vi "servo chB.vi"(0 "Servo Position (0 - 255)":u8(slide)=128 step=1 scale=0.0..255.0, 1 "Controller Daisy Chain Position (1 - 4)":u8=1, 4 "Enable Sync: Fast | Medium | Slow | None":string(combo)="None", 5 "Select Servo":string(combo)="Servo 1", 6 "Enum":enum16{"A", "B"}(ring), 7 "error in (no error)":errorcluster) -> (2 "error out":errorcluster)   [LabVIEW 2018]
uses:
  <vilib>/myRIO/Instrument Drivers/Onboard IO/I2C/typedefs/I2C User Configuration.ctl
  <vilib>/myRIO/Instrument Drivers/Onboard IO/I2C/typedefs/I2C Transfer Rate.ctl
  <vilib>/myRIO/Instrument Drivers/Onboard IO/I2C/typedefs/I2C Reference.ctl
  <vilib>/myRIO/Common/Instrument Driver Framework/Utilities/typedefs/myRIO Generic Hardware Reference.ctl
  <vilib>/myRIO/Common/Instrument Driver Framework/Utilities/typedefs/Hardware Version Enum.ctl
  <vilib>/myRIO/Common/Instrument Driver Framework/Utilities/typedefs/myRIO v1.0 Reference.ctl
  <vilib>/myRIO/Common/Instrument Driver Framework/Utilities/typedefs/Generic FPGA Reference.ctl
  <vilib>/myRIO/Common/Instrument Driver Framework/myRIO v1.0/I2C/typedefs/I2C Channels Enum.ctl
  <vilib>/myRIO/Instrument Drivers/Onboard IO/I2C/typedefs/I2C Configuration.ctl
  <vilib>/userdefined/High Color/nirio_resource_hc.ctl
  <vilib>/myRIO/Common/Instrument Driver Framework/Utilities/vis/Is FPGA Ref Available.vi
  <vilib>/myRIO/Common/Instrument Driver Framework/myRIO v1.0/I2C/vis/myRIO v1.1 Open I2C.vi
  <vilib>/myRIO/Instrument Drivers/Onboard IO/I2C/vis/Configure.vi
  <vilib>/myRIO/Instrument Drivers/Onboard IO/I2C/vis/Write.vi
  <vilib>/myRIO/Common/Instrument Driver Framework/Utilities/vis/Validate Channels.vi
  <vilib>/myRIO/Common/Instrument Driver Framework/myRIO v1.0/I2C/vis/myRIO v1.0 Reserve I2C.vi
  <vilib>/myRIO/Common/Instrument Driver Framework/myRIO v1.0/I2C/vis/myRIO v1.0 Build MUX Configuration I2C.vi
  <vilib>/myRIO/Common/Instrument Driver Framework/myRIO v1.0/Resource Manager/vis/myRIO v1.0 Reserve Channel List.vi
  <vilib>/myRIO/Common/Instrument Driver Framework/myRIO v1.0/Resource Manager/vis/myRIO v1.0 Create Configuration List.vi
  <vilib>/myRIO/Common/Instrument Driver Framework/myRIO v1.0/Resource Manager/vis/myRIO v1.0 Reserve Channel.vi
  <vilib>/myRIO/Common/Instrument Driver Framework/myRIO v1.0/Resource Manager/vis/myRIO v1.0 Unreserve Channel.vi
  <vilib>/myRIO/Common/Instrument Driver Framework/myRIO v1.0/Resource Manager/vis/myRIO v1.0 Build Mutex Name.vi
  <vilib>/Utility/VariantDataType/GetNumericInfo.vi
  <vilib>/Utility/error.llb/Error Cluster From Error Code.vi
  <vilib>/myRIO/Common/Instrument Driver Framework/myRIO v1.0/myRIO v1.1 Open.vi
  <vilib>/myRIO/Common/Instrument Driver Framework/Utilities/vis/IO Manager.vi
  <vilib>/myRIO/Common/Instrument Driver Framework/Utilities/vis/Configuration Manager.vi
  <vilib>/myRIO/Common/Instrument Driver Framework/myRIO v1.0/Resource Manager/vis/myRIO v1.0 Configure IO.vi
  <vilib>/myRIO/Common/Instrument Driver Framework/myRIO v1.0/myRIO v1.0 Close.vi
  <vilib>/myRIO/Common/Instrument Driver Framework/myRIO v1.0/I2C/vis/myRIO v1.0 Configure I2C.vi
  <vilib>/myRIO/Common/Instrument Driver Framework/myRIO v1.0/I2C/vis/myRIO v1.0 Write I2C.vi
  <vilib>/myRIO/Express VI/Onboard IO/I2C/I2C Express VI.xnode
  <vilib>/myRIO/Instrument Drivers/Onboard IO/I2C/vis/myRIO I2C Open.xnode
  <vilib>/myRIO/Instrument Drivers/Onboard IO/I2C/I2C.lvlib
panel:
  out "error out 2":errorcluster
  in  "error in (no error) 2":errorcluster
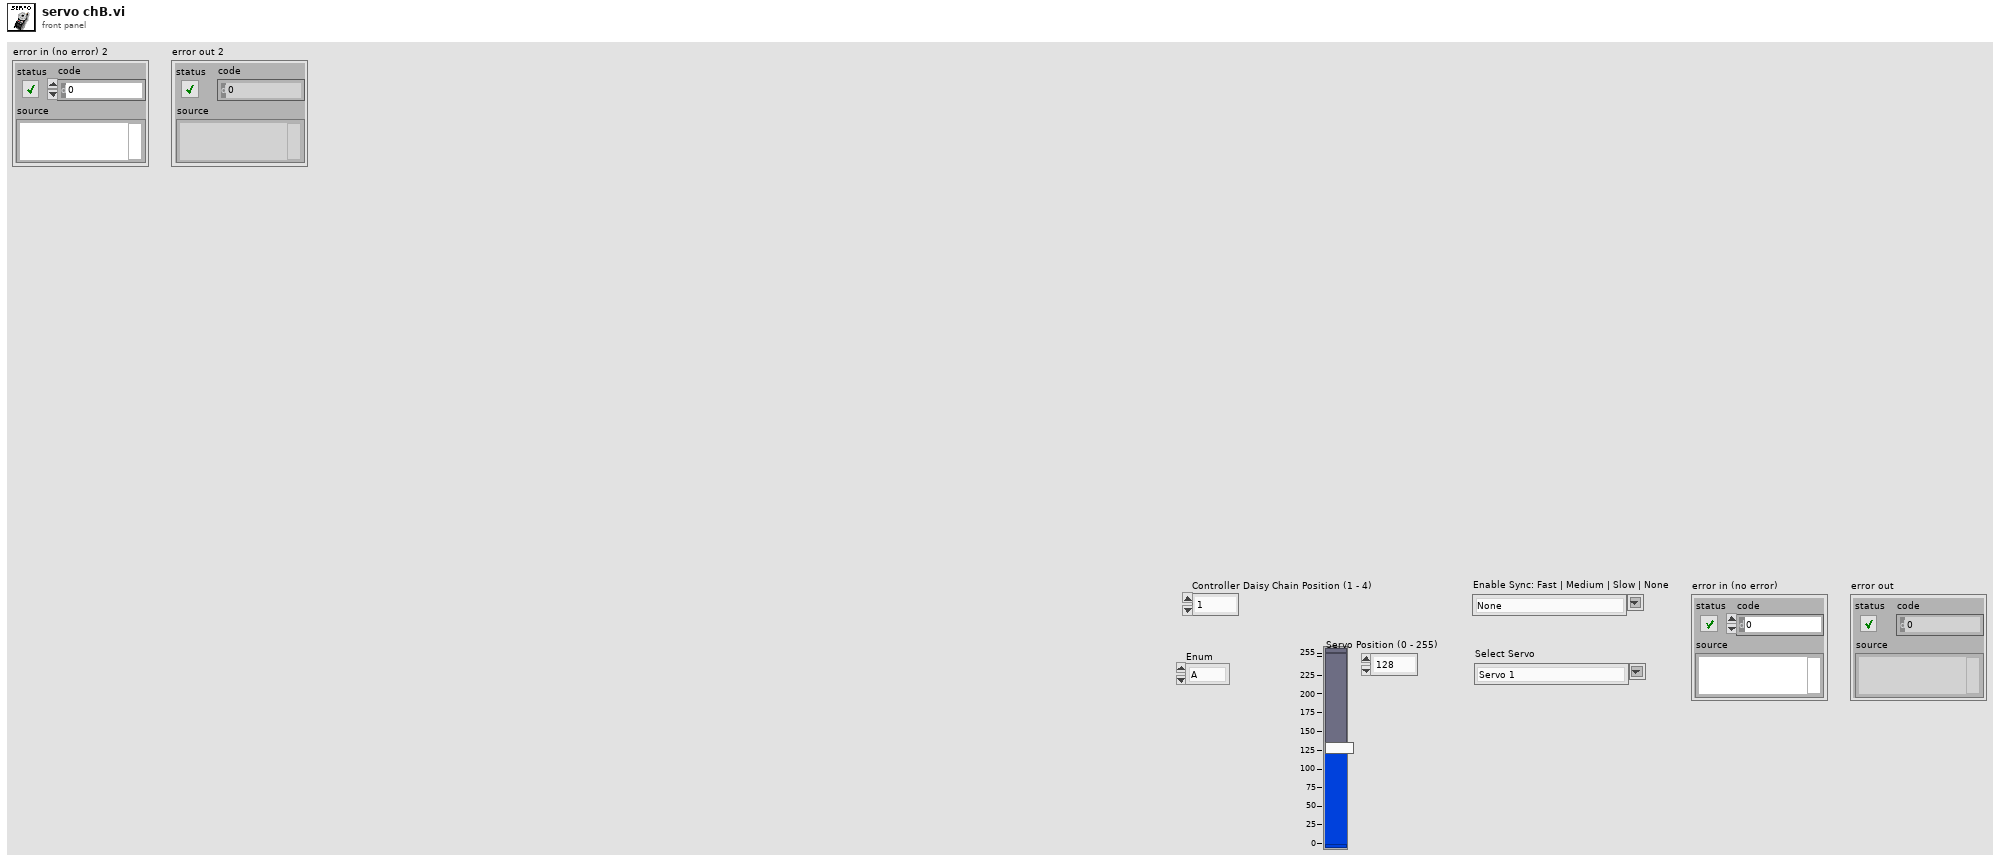
[diagram p1: front panel]
types:
  T1 = typedef "I2C.lvlib/I2C Reference.ctl" = cluster{"myRIO Reference":T2, "I2C Channels Enum":T6, "I2C Configuration":T7}
  T2 = typedef "myRIO Generic Hardware Reference.ctl" = cluster{"myRIO Model":T3, "myRIO Hardware Reference":T4}
  T3 = typedef "Hardware Version Enum.ctl" = enum16{"Unknown", "myRIO-1900", "myRIO-1950", "roboRIO", "NI ELVIS RIO CM", "ELVIS III"}
  T4 = typedef "myRIO v1.0 Reference.ctl" = cluster{"Generic FPGA Reference":T5, "Allow multiple opens":bool}
  T5 = typedef "Generic FPGA Reference.ctl" = refnum<k20>
  T6 = typedef "I2C Channels Enum.ctl" = enum16{"Not Connected", "A/I2C", "B/I2C", "I2C/I2C"}
  T7 = typedef "I2C.lvlib/I2C Configuration.ctl" = cluster{"I2C Transfer Rate":T8}
  T8 = typedef "I2C.lvlib/I2C Transfer Rate.ctl" = enum16{"Standard mode (100 kbps)", "Fast mode (400 kbps)"}
  T9 = typedef "I2C.lvlib/I2C User Configuration.ctl" = cluster{"I2C Transfer Rate":T8}
  T10 = typedef "nirio_resource_hc.ctl" = tag
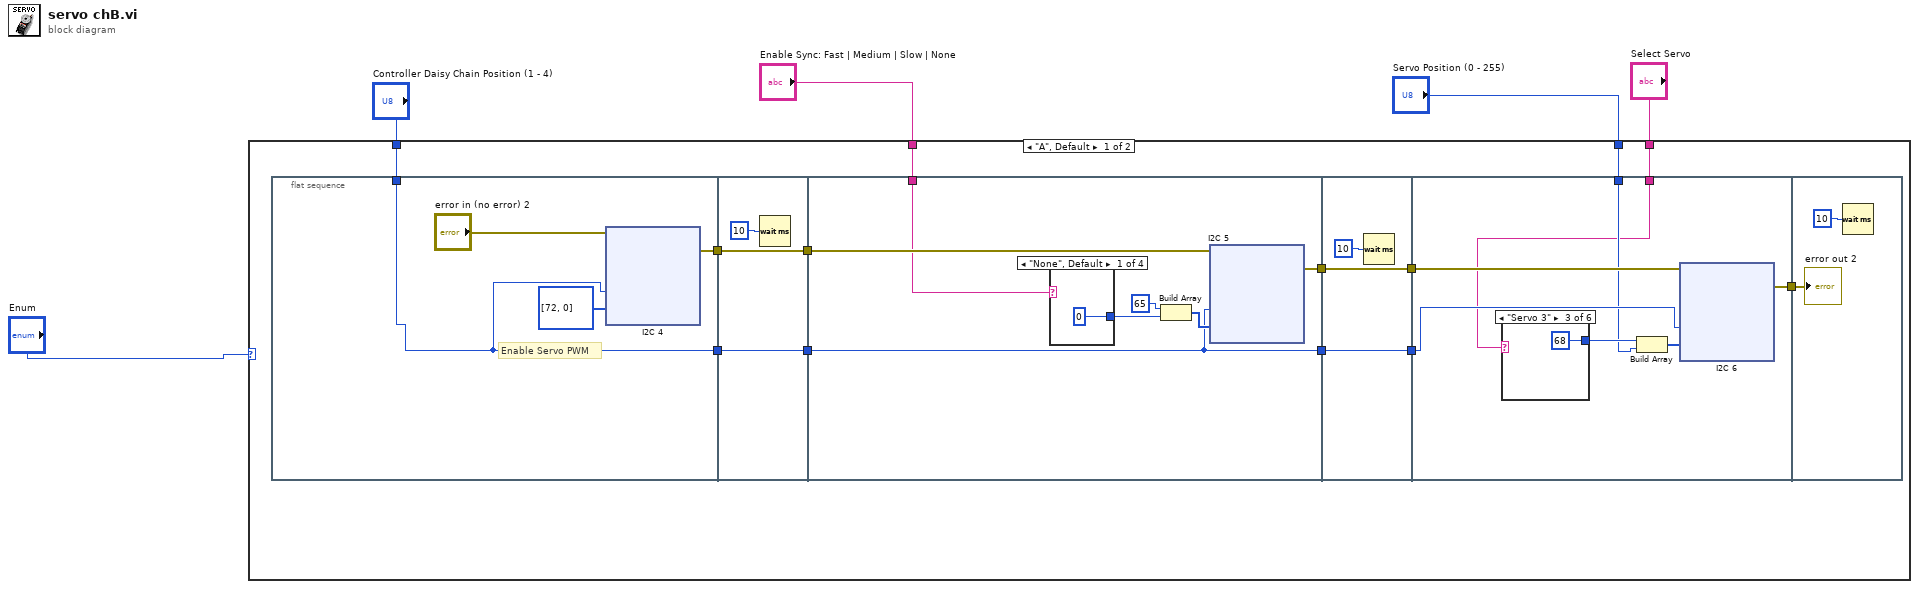
[diagram p0: block diagram]
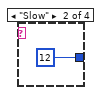
[diagram p2: hidden frame]
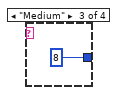
[diagram p3: hidden frame]
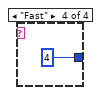
[diagram p4: hidden frame]
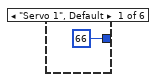
[diagram p5: hidden frame]
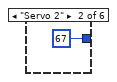
[diagram p6: hidden frame]
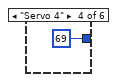
[diagram p7: hidden frame]
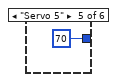
[diagram p8: hidden frame]
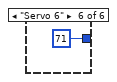
[diagram p9: hidden frame]
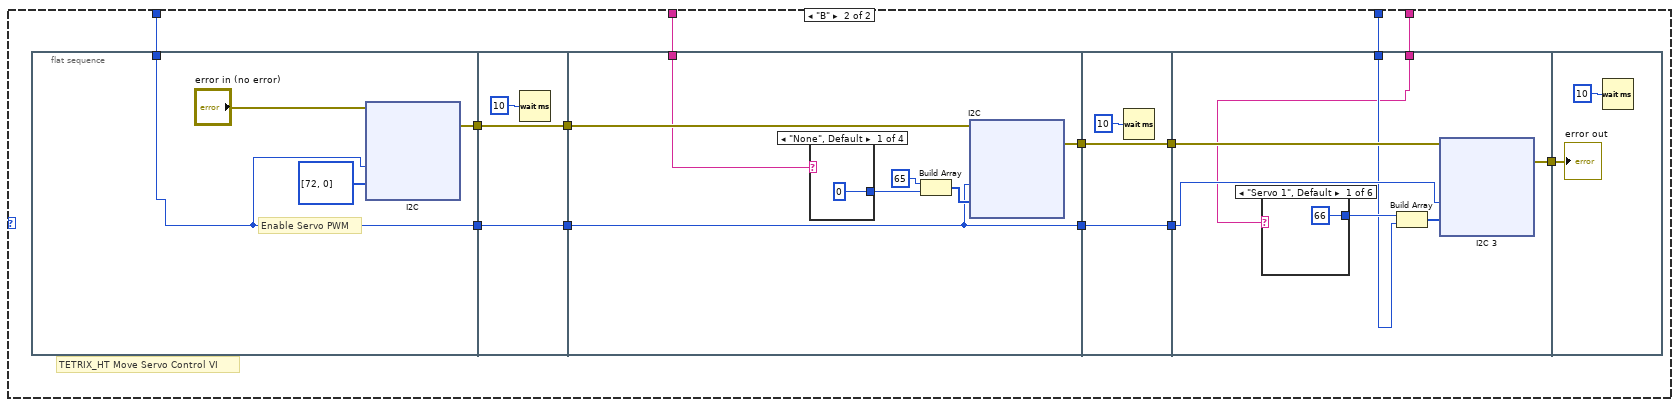
[diagram p10: hidden frame]
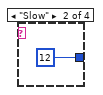
[diagram p11: hidden frame]
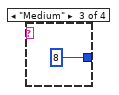
[diagram p12: hidden frame]
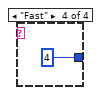
[diagram p13: hidden frame]
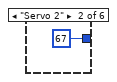
[diagram p14: hidden frame]
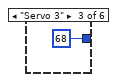
[diagram p15: hidden frame]
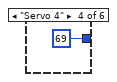
[diagram p16: hidden frame]
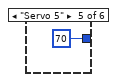
[diagram p17: hidden frame]
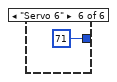
[diagram p18: hidden frame]
diagram:
  n1 = case shown="\"A\", Default" "Enum" {
    tunnel: "Servo Position (0 - 255)" -> [w7 w172]
    tunnel: "Enable Sync: Fast | Medium | Slow | None" -> [w8 w171]
    tunnel: "Controller Daisy Chain Position (1 - 4)" -> [w9 w170]
    tunnel: "Select Servo" -> [w6 w169]
    frame "A", Default {
      n2 = flat-sequence {
        tunnel: [w19] -> w18
        tunnel: [w21] -> w17
        tunnel: w9 -> [w19]
        tunnel: w18 -> [w63]
        tunnel: [w63] -> w16
        tunnel: w17 -> [w62]
        tunnel: [w62] -> w15
        tunnel: [w67] -> w14
        tunnel: w16 -> [w65]
        tunnel: w15 -> [w66]
        tunnel: [w65] -> w13
        tunnel: w8 -> [w64]
        tunnel: w14 -> [w115]
        tunnel: [w115] -> w12
        tunnel: w13 -> [w114]
        tunnel: [w114] -> w11
        tunnel: w12 -> [w119]
        tunnel: w11 -> [w120]
        tunnel: [w118] -> w10
        tunnel: w7 -> [w117]
        tunnel: w6 -> [w116]
        tunnel: w10 -> [w167]
        frame #0 {
          # "Enable Servo PWM"
          n3 = xnode "I2C 4"("Slave Address (7-bit)"=w19, "Bytes to Write"=u8[] [72, 0], "error in (no error)"="error in (no error) 2") -> ("error out"=w21:errorcluster)
        }
        frame #1 {
          n4 = Wait (ms)(milliseconds to wait=u32 10) -> ()  [unwired: 1 out]
        }
        frame #2 {
          n5 = case shown="\"None\", Default" w64 {
            tunnel: [u8 0 u8 12 u8 8 u8 4] -> w68
            frame "None", Default {
            }
            frame "Slow" {
            }
            frame "Medium" {
            }
            frame "Fast" {
            }
          }
          n6 = Build Array(u8 65 ("element"), w68) -> (w69:u8[])
          n7 = xnode "I2C 5"("Slave Address (7-bit)"=w65, "Bytes to Write"=w69, "error in (no error)"=w66) -> ("error out"=w67:errorcluster)
        }
        frame #3 {
          n8 = Wait (ms)(milliseconds to wait=u32 10) -> ()  [unwired: 1 out]
        }
        frame #4 {
          n9 = case shown="\"Servo 3\"" w116 {
            tunnel: [u8 66 u8 67 u8 68 u8 69 u8 70 u8 71] -> w122
            frame "Servo 1", Default {
            }
            frame "Servo 2" {
            }
            frame "Servo 3" {
            }
            frame "Servo 4" {
            }
            frame "Servo 5" {
            }
            frame "Servo 6" {
            }
          }
          n10 = Build Array(w122, w117) -> (w121:u8[])
          n11 = xnode "I2C 6"("Slave Address (7-bit)"=w120, "Bytes to Write"=w121, "error in (no error)"=w119) -> ("error out"=w118:errorcluster)
        }
        frame #5 {
          n12 = Wait (ms)(milliseconds to wait=u32 10) -> ()  [unwired: 1 out]
          "error out 2" <- w167
        }
      }
    }
    frame "B" {
      # "TETRIX_HT Move Servo Control VI"
      n13 = flat-sequence {
        tunnel: [w182] -> w181
        tunnel: [w184] -> w180
        tunnel: w170 -> [w182]
        tunnel: w181 -> [w226]
        tunnel: [w226] -> w179
        tunnel: w180 -> [w225]
        tunnel: [w225] -> w178
        tunnel: [w230] -> w177
        tunnel: w179 -> [w228]
        tunnel: w178 -> [w229]
        tunnel: [w228] -> w176
        tunnel: w171 -> [w227]
        tunnel: w177 -> [w278]
        tunnel: [w278] -> w175
        tunnel: w176 -> [w277]
        tunnel: [w277] -> w174
        tunnel: w175 -> [w282]
        tunnel: w174 -> [w283]
        tunnel: [w281] -> w173
        tunnel: w172 -> [w280]
        tunnel: w169 -> [w279]
        tunnel: w173 -> [w330]
        frame #0 {
          # "Enable Servo PWM"
          n14 = xnode "I2C"("Slave Address (7-bit)"=w182, "Bytes to Write"=u8[] [72, 0], "error in (no error)"="error in (no error)") -> ("error out"=w184:errorcluster)
        }
        frame #1 {
          n15 = Wait (ms)(milliseconds to wait=u32 10) -> ()  [unwired: 1 out]
        }
        frame #2 {
          n16 = case shown="\"None\", Default" w227 {
            tunnel: [u8 0 u8 12 u8 8 u8 4] -> w231
            frame "None", Default {
            }
            frame "Slow" {
            }
            frame "Medium" {
            }
            frame "Fast" {
            }
          }
          n17 = Build Array(u8 65 ("element"), w231) -> (w232:u8[])
          n18 = xnode "I2C"("Slave Address (7-bit)"=w228, "Bytes to Write"=w232, "error in (no error)"=w229) -> ("error out"=w230:errorcluster)
        }
        frame #3 {
          n19 = Wait (ms)(milliseconds to wait=u32 10) -> ()  [unwired: 1 out]
        }
        frame #4 {
          n20 = case shown="\"Servo 1\", Default" w279 {
            tunnel: [u8 66 u8 67 u8 68 u8 69 u8 70 u8 71] -> w285
            frame "Servo 1", Default {
            }
            frame "Servo 2" {
            }
            frame "Servo 3" {
            }
            frame "Servo 4" {
            }
            frame "Servo 5" {
            }
            frame "Servo 6" {
            }
          }
          n21 = Build Array(w285, w280) -> (w284:u8[])
          n22 = xnode "I2C 3"("Slave Address (7-bit)"=w283, "Bytes to Write"=w284, "error in (no error)"=w282) -> ("error out"=w281:errorcluster)
        }
        frame #5 {
          n23 = Wait (ms)(milliseconds to wait=u32 10) -> ()  [unwired: 1 out]
          "error out" <- w330
        }
      }
    }
  }
